vi "Login.vi"   [LabVIEW 2009, in "Vertical Turbine.lvlib"]
doc: "Used in the demonstration of namespacing and access scope of general project libraries. Users should note that XControls and Classes are specific types of project libraries.\n\nAAL 9/09"
uses:
  Vertical Turbine.lvlib
panel:
  # "Login for Vertical Wind Turbine"
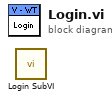
[diagram p0: block diagram]
diagram:
  n1 = call "Login SubVI.vi"() -> ()  [unwired: 1 out]
